vi "database path.vi"(10 "ping":bool, 11 "database":string="database1") -> (2 "Connection information":string, 3 "Path out":string)   [LabVIEW 2016]
uses:
  Access/Access Lib.lvlib
  SQLite/SQLite Lib.lvlib
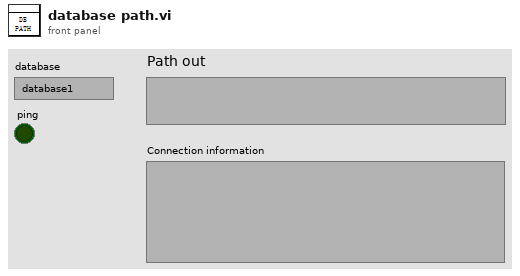
[diagram p1: front panel]
types:
  T1 = typedef "数据库类型.ctl" = enum16{"Access", "SQLite"}
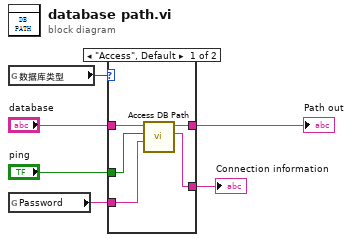
[diagram p0: block diagram]
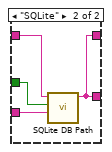
[diagram p2: hidden frame]
diagram:
  n1 = global read "外部调用接口全局变量.vi" "数据库类型"() -> (w1:T1)
  n2 = global read "外部调用接口全局变量.vi" "Password"() -> (w2:string)
  n3 = case shown="\"Access\", Default" w1 {
    tunnel: [w11 w13] -> w4
    tunnel: "database" -> [w10 w15]
    tunnel: "ping" -> [w9 w14]
    tunnel: [w8 w13] -> w3
    tunnel: w2 -> [w7 w12]
    frame "Access", Default {
      n4 = call "Access DB Path.vi"("Password"=w7, "ping"=w9, "database"=w10) -> ("Connection information"=w8:string, "Path out"=w11:string)  [unwired: 7 in]
    }
    frame "SQLite" {
      n5 = call "SQLite DB Path.vi"("Password"=w12, "ping"=w14, "database"=w15) -> ("Path out"=w13:string)  [unwired: 8 in]
    }
  }
  "Path out" <- w4
  "Connection information" <- w3
